vi "Send Count Down Finished.vi"(8 "error in (no error)":errorcluster, 11 "Timer Actor in":refnum<class "Timer Actor.lvclass">) -> (0 "error out":errorcluster, 3 "Timer Actor out":refnum<class "Timer Actor.lvclass">)   [LabVIEW 2024, in "Timer Actor.lvlib" / "Timer Actor.lvclass"]
uses:
  Timer Actor.lvclass
  <vilib>/ActorFramework/Actor/Actor.lvclass/Actor.ctl
  Chef States Logic/Chef States Logic Messages/Update State String Msg/Update State String Msg.lvclass/Update State String Msg.ctl
  <vilib>/ActorFramework/Message Enqueuer/Message Enqueuer.lvclass/Message Enqueuer.ctl
  <vilib>/ActorFramework/Message Enqueuer/Enqueue.vi
  Chef States Logic/Chef States Logic Messages/Update State String Msg/Update State String Msg.lvclass
  <vilib>/ActorFramework/Message Priority Queue/Priority Enqueue.vi
  Timer Actor.lvclass/Timer Actor.ctl
  <vilib>/ActorFramework/Actor/Actor.lvclass
  Cooker Actor/Cooker Actor Messages/Update Kitchen Table Step Done by Index Msg/Update Kitchen Table Step Done by Index Msg.lvclass
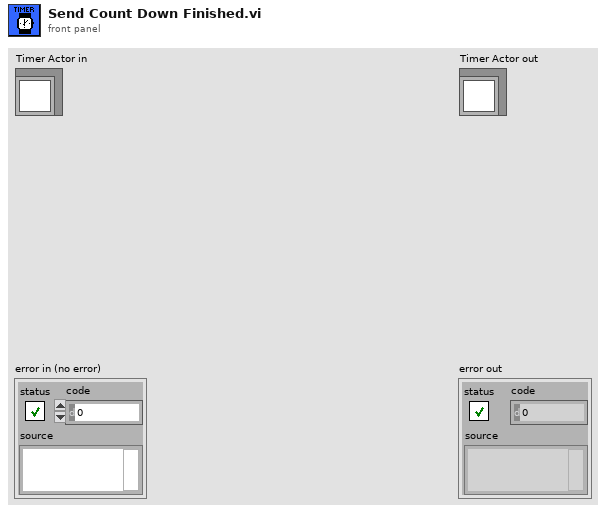
[diagram p1: front panel]
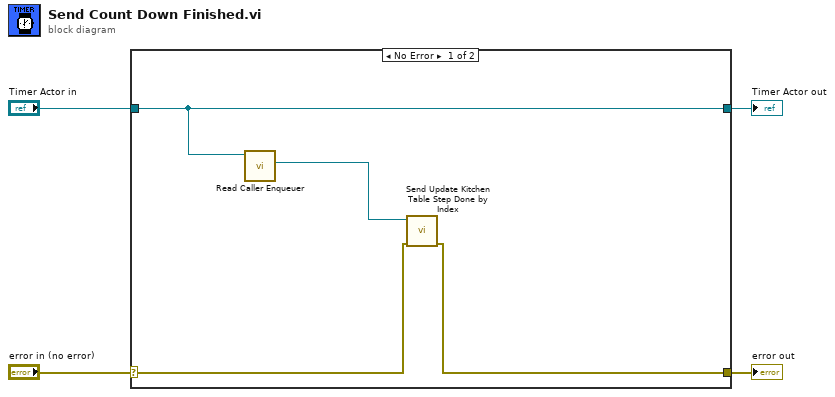
[diagram p0: block diagram]
diagram:
  n1 = case shown="No Error" "error in (no error)" {
    selector: "error in (no error)" -> [w7 w10]
    tunnel: [w6 w10] -> w3
    tunnel: [w8 w9] -> w1
    tunnel: "Timer Actor in" -> [w8 w9]
    frame No Error {
      n2 = call <vilib>:"Read Caller Enqueuer.vi"("Actor"=w8) -> ("Caller Enqueuer"=w5:refnum<class "Message Enqueuer.lvclass">)  [unwired: 10 in]
      n3 = call "Send Update Kitchen Table Step Done by Index.vi"("error in (no error)"=w7, "Message Enqueuer"=w5) -> ("error out"=w6:errorcluster)  [unwired: 8 in, 1 out]
    }
    frame Error {
    }
  }
  "error out" <- w3
  "Timer Actor out" <- w1
